vi "Configure Trigger.vi"(6 "Trigger Source (0: Immediate)":i32(ring) items=["Immediate", "External", "Bus"], 7 "Slop (1: Negative)":i32(ring)=1 items=["Positive", "Negative"], 8 "error in (no error)":errorcluster, 9 "Delay Time (0 s)":dbl, 10 "Trigger Counter (1)":dbl=1.0, 11 "VISA resource name":refnum<visa-resource-name>) -> (0 "error out":errorcluster, 3 "VISA resource name out":refnum<visa-resource-name>)   [LabVIEW 2021, in "Agilent 532XX Series.lvlib"]
doc: "Configures the characteristics of the trigger system."
uses:
  <instrlib>/Agilent 532XX Series/Agilent 532XX Series.lvlib
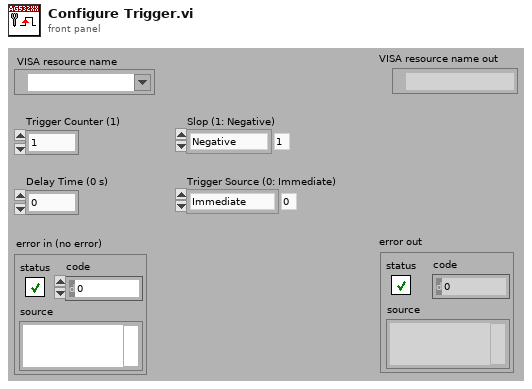
[diagram p1: front panel]
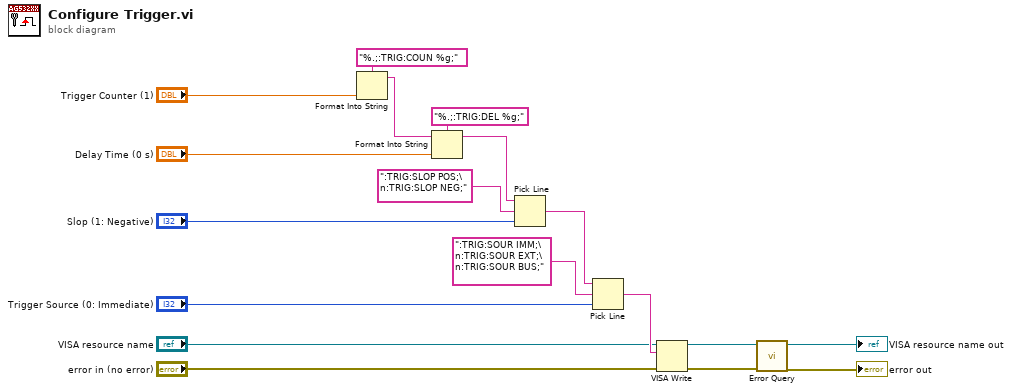
[diagram p0: block diagram]
diagram:
  n1 = Format Into String(format string="%.;:TRIG:COUN %g;", "Trigger Counter (1)") -> (resulting string=w16:string)  [unwired: 2 in, 1 out]
  n2 = Format Into String(format string="%.;:TRIG:DEL %g;", initial string=w16, "Delay Time (0 s)") -> (resulting string=w11:string)  [unwired: 1 in, 1 out]
  n3 = Pick Line(string ("")=w11, multi-line string=":TRIG:SLOP POS;\n:TRIG:SLOP NEG;", line index="Slop (1: Negative)") -> (output string=w8:string)
  n4 = Pick Line(string ("")=w8, multi-line string=":TRIG:SOUR IMM;\n:TRIG:SOUR EXT;\n:TRIG:SOUR BUS;", line index="Trigger Source (0: Immediate)") -> (output string=w7:string)
  n5 = VISA Write(VISA resource name="VISA resource name", write buffer=w7, error in (no error)="error in (no error)") -> (VISA resource name out=w4:refnum<visa-resource-name>, error out=w3:errorcluster)  [unwired: 1 out]
  n6 = call <instrlib>:"Error Query.vi"("error in (no error)"=w3, "VISA resource name"=w4) -> ("error out"=→"error out":errorcluster, "VISA resource name out"=→"VISA resource name out":refnum<visa-resource-name>)  [unwired: 8 out]
